vi "Ke2400 VI Controler.vi"(5 "ON/OFF":bool=TRUE, 6 "Curr Range":dbl=0.01, 7 "Voltage Range":i32=100, 8 "error in (no error)":errorcluster, 9 "Idd Compliace(mA)":dbl=6.0, 10 "Volt Level":dbl, 11 "VISA In":refnum<visa-resource-name>) -> (0 "error out":errorcluster, 3 "VISA Out":refnum<visa-resource-name>)   [LabVIEW 2012]
doc: "This VI is to setup IV before Measuring\nCurr Range default = 0\nCurr Compliance = 6uA\nVoltage Range = 100V\nVoltage level = 0V\nBy default is ON"
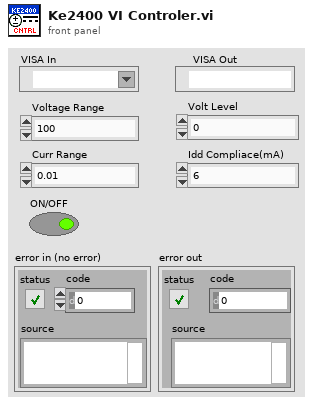
[diagram p1: front panel]
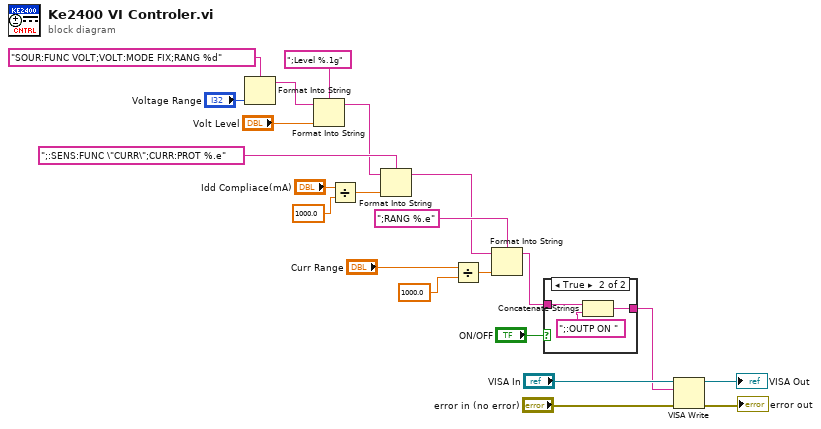
[diagram p0: block diagram]
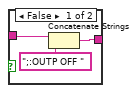
[diagram p2: hidden frame]
diagram:
  n1 = Format Into String(format string="SOUR:FUNC VOLT;VOLT:MODE FIX;RANG %d", "Voltage Range") -> (resulting string=w7:string)  [unwired: 2 in, 1 out]
  n2 = Format Into String(format string=";Level %.1g", initial string=w7, "Volt Level") -> (resulting string=w4:string)  [unwired: 1 in, 1 out]
  n3 = Divide(x="Idd Compliace(mA)", y=1000.0) -> (x/y=w18:dbl)
  n4 = Format Into String(format string=";:SENS:FUNC \"CURR\";CURR:PROT %.e", initial string=w4, w18) -> (resulting string=w8:string)  [unwired: 1 in, 1 out]
  n5 = Divide(x="Curr Range", y=1000.0) -> (x/y=w13:dbl)
  n6 = Format Into String(format string=";RANG %.e", initial string=w8, w13) -> (resulting string=w2:string)  [unwired: 1 in, 1 out]
  n7 = case shown="True" "ON/OFF" {
    tunnel: w2 -> [w24 w27]
    tunnel: [w23 w26] -> w1
    frame False {
      n8 = Concatenate Strings(w24, ";:OUTP OFF " ("format string")) -> (w23:string)
    }
    frame True {
      n9 = Concatenate Strings(w27, ";:OUTP ON " ("format string")) -> (w26:string)
    }
  }
  n10 = VISA Write(VISA resource name="VISA In", write buffer=w1, error in (no error)="error in (no error)") -> (VISA resource name out=→"VISA Out":refnum<visa-resource-name>, error out=→"error out":errorcluster)  [unwired: 1 out]
